vi "calibrateRefMicro.vi"(8 "error in (no error)":errorcluster, 9 "enable IEPE excitation (F)":bool, 10 "DAQmx physical channel":tag="SOUNDACQ/ai1", 11 "calibration settings":T5={"calibration value [dB SPL]"=114.0, "calibration frequency [Hz]"=1000.0}) -> (0 "error out":errorcluster, 2 "power spectrum":cluster{"x0":dbl, "dx":dbl, "magnitude":dbl[]}(graph), 3 "calibrated sensor sensitivity [mV/Pa]":dbl=nan format="%.2g")   [LabVIEW 2018]
uses:
  <vilib>/addons/_NISVFA/_Shared subVIs/Controls/svc_Channel Info.ctl
  <vilib>/addons/_NISVFA/_Shared subVIs/Controls/svc_Engineering Units Text Ring.ctl
  <vilib>/addons/_NISVFA/_Shared subVIs/Controls/svc_Weighting Filter Text Ring.ctl
  <vilib>/addons/Sound and Vibration/svt_Calibration/SoundVib_Calibration.lvlib
panel:
  out "calibrated channel info":T1={"sensor sensitivity"=nan, "engineering units"=2, "dB reference"=2e-05, "custom label"="EU", "weighting filter"=0, "pregain"=0.0} {"pregain" format="%.2f"; "weighting filter" items=["Linear", "A-weighting", "B-weighting", "C-weighting", "ITU-R 468-4", "Dolby", "CCITT", "C-message", "Wb", "Wc", "Wd", "We", "Wf", "Wh", "Wj", "Wk", "Wm", "AES17 20 kHz lowpass", "AES17 40 kHz lowpass", "AES17 20 kHz highpass", "AES17 40 kHz highpass"]; "dB reference" format="%^.1e"; "engineering units" items=["custom..."=0, "V"=1, "A"=21, "C"=30, "pC"=31, "s"=32, "-"=29, "Pa"=2, "N"=20, "g"=3, "m/s^2"=4, "m/s"=5, "m"=6, "mm/s"=12, "mm"=13, "micron/s"=14, "micron"=15, "in/s^2"=7, "in/s"=8, "in"=9, "mil/s"=10, "mil"=11, "rad/s^2"=16, "rad/s"=17, "rad"=18, "deg/s^2"=26, "deg/s"=27, "deg"=28, "RPM"=22, "cycle/s^2"=23, "Hz"=24, "cycle"=25, "strain"=19]; "sensor sensitivity" format="%#_5f"}
  in  "channel configuration":T4={"maximum value (V)"=0.3, "minimum value (V)"=-0.3, "terminal configuration"=-1} {"terminal configuration" items=["Default"=-1, "RSE"=10083, "NRSE"=10078, "Differential"=10106, "Pseudodifferential"=12529]}
  out "frequency [Hz]":dbl=nan format="%.2f"
  out "amplitude [V rms]":dbl=nan format="%.4f"
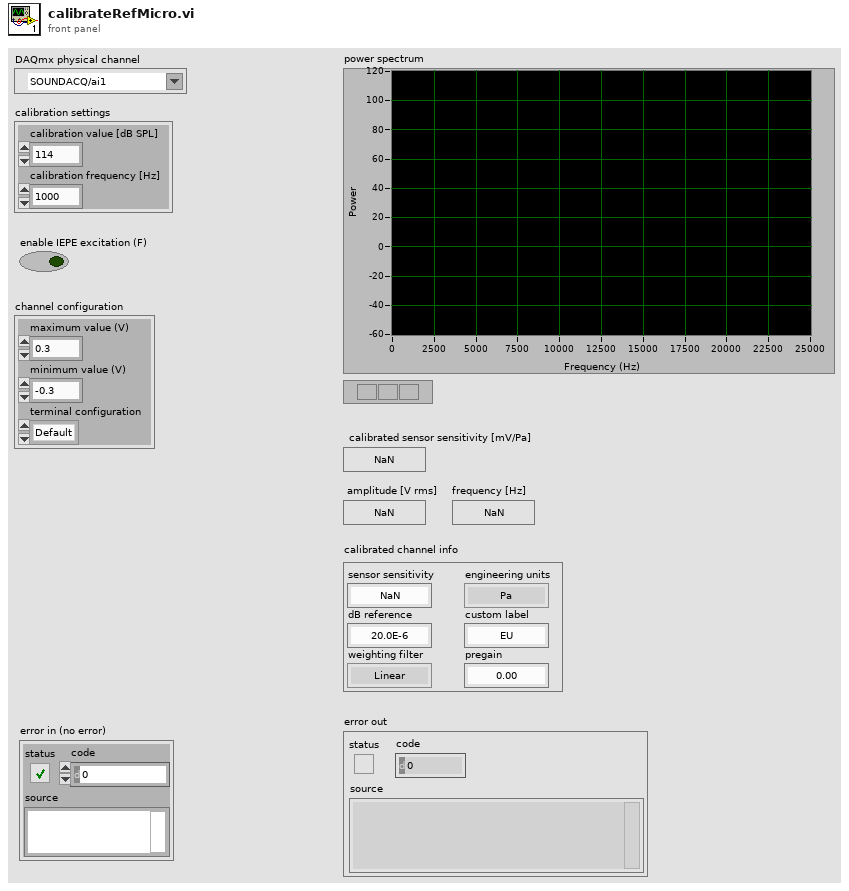
[diagram p1: front panel]
types:
  T1 = typedef "svc_Channel Info.ctl" = cluster{"sensor sensitivity":dbl, "engineering units":T2, "dB reference":dbl, "custom label":string, "weighting filter":T3, "pregain":dbl}
  T2 = typedef "svc_Engineering Units Text Ring.ctl" = u16
  T3 = typedef "svc_Weighting Filter Text Ring.ctl" = u16
  T4 = cluster{"maximum value (V)":dbl, "minimum value (V)":dbl, "terminal configuration":i32}
  T5 = cluster{"calibration value [dB SPL]":dbl, "calibration frequency [Hz]":dbl}
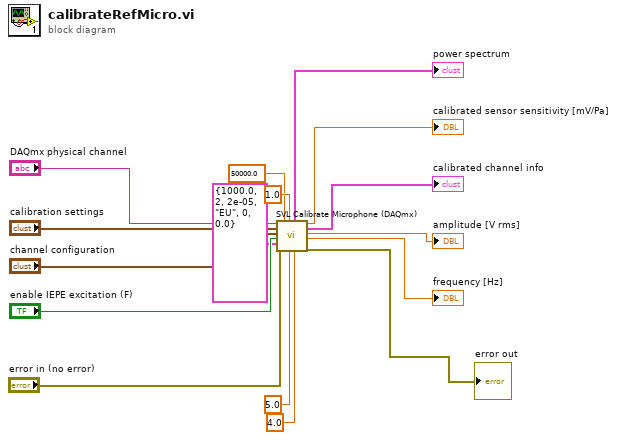
[diagram p0: block diagram]
diagram:
  n1 = call <vilib>:"SVL Calibrate Microphone (DAQmx).vi"("DAQmx physical channel"="DAQmx physical channel", "calibration settings"="calibration settings", "channel configuration"="channel configuration", "enable IEPE excitation (F)"="enable IEPE excitation (F)", "channel info"=T1 {"sensor sensitivity"=1000.0, "engineering units"=2, "dB reference"=2e-05, "custom label"="EU", "weighting filter"=0, "pregain"=0.0}, "error in (no error)"="error in (no error)", "sampling frequency [Hz]"=50000.0, "duration [s]"=1.0, "time to settle [s]"=5.0, "IEPE current [mA]"=4.0) -> ("power spectrum"=→"power spectrum":cluster{"x0":dbl, "dx":dbl, "magnitude":dbl[]}, "calibrated sensor sensitivity [mV/Pa]"=→"calibrated sensor sensitivity [mV/Pa]":dbl, "calibrated channel info"=→"calibrated channel info":T1, "amplitude [V rms]"=→"amplitude [V rms]":dbl, "frequency [Hz]"=→"frequency [Hz]":dbl, "error out"=→"error out":errorcluster)  [unwired: 3 in, 1 out]
